vi "automatic_feeder.vi"() -> ()   [LabVIEW 2017]
panel:
  out "Boolean":bool
  out "Low  2":bool
  out "Ok  2":bool
  out "Full  2":bool
  out "Cup 2":dbl(slide) scale=0.0..3.0
  out "Tank 2":dbl(slide)=6.0 scale=0.0..3.0
  out "Lamp":bool
  in  "Thermometer":i32(slide) scale=0.0..100.0
  in  "Reset":bool
  in  "Lamp":bool
  in  "Stop":bool
  in  "?":bool
  out "Low":bool
  out "Ok":bool
  out "Full":bool
  out "Tank":dbl(slide)=6.0 scale=0.0..5.0
  out "Cup":dbl(slide) scale=0.0..5.0
  out "OK Button":bool
  in  "Clock":i32(knob)=1 min=1 max=12 scale=1.0..12.0
  # "EMPTY/FILL"
  # "FOOD"
  # "WATER"
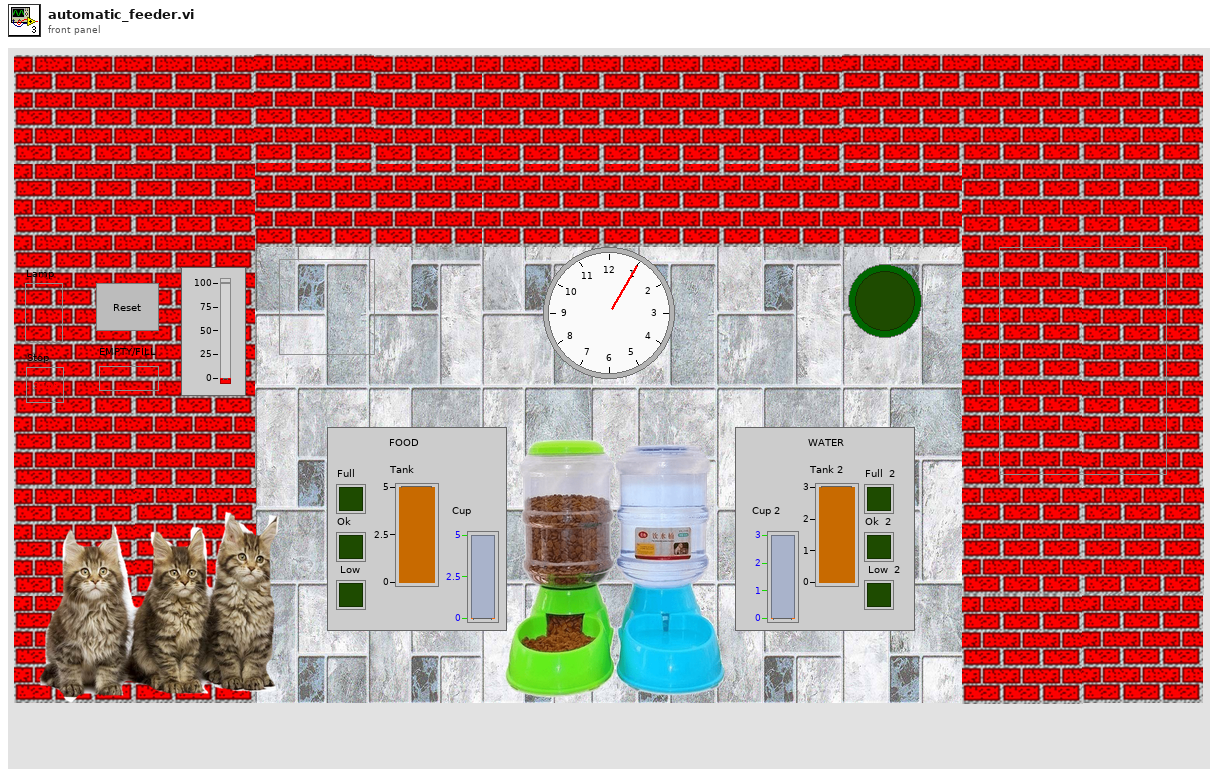
[diagram p1: front panel]
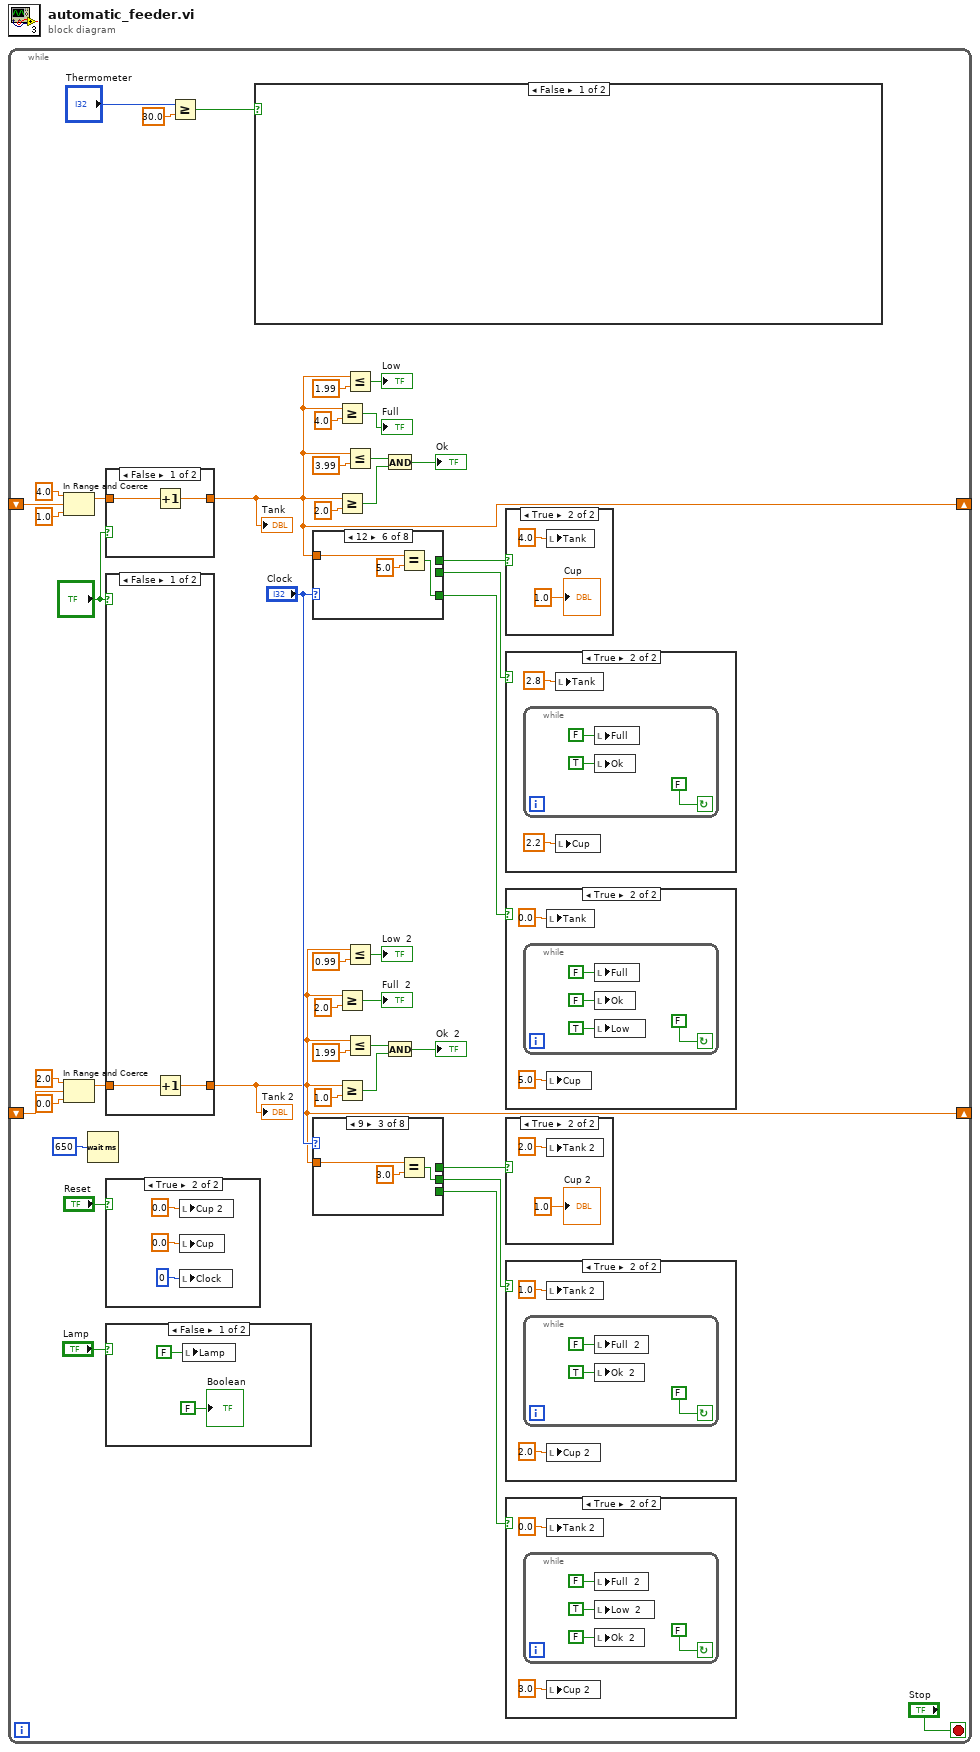
[diagram p0: block diagram]
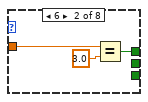
[diagram p6: hidden frame]
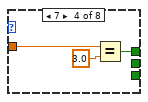
[diagram p7: hidden frame]
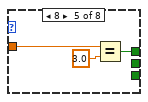
[diagram p8: hidden frame]
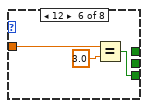
[diagram p9: hidden frame]
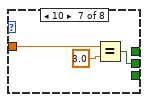
[diagram p10: hidden frame]
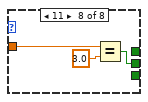
[diagram p11: hidden frame]
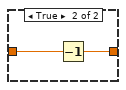
[diagram p12: hidden frame]
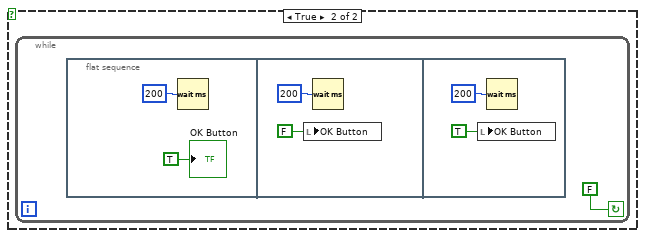
[diagram p13: hidden frame]
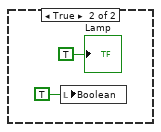
[diagram p14: hidden frame]
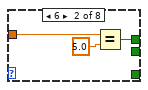
[diagram p19: hidden frame]
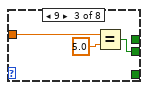
[diagram p20: hidden frame]
diagram:
  n1 = while {
    shift-right: [w27] -> _
    shift-left: _ -> [w30]
    shift-right: [w8] -> _
    shift-left: _ -> [w19]
    stop <- "Stop" stop-if-true
    n2 = In Range and Coerce(upper limit=4.0, x=w30, lower limit=1.0) -> (coerced(x)=w40:dbl)  [unwired: 1 out]
    n3 = In Range and Coerce(upper limit=2.0, x=w19, lower limit=0.0) -> (coerced(x)=w16:dbl)  [unwired: 1 out]
    n4 = Wait (ms)(milliseconds to wait=u32 650) -> ()  [unwired: 1 out]
    n5 = case shown="False" "?" {
      tunnel: w40 -> [w131 w133]
      tunnel: [w130 w132] -> w27
      frame False {
        n6 = Increment(x=w131) -> (x+1=w130:dbl)
      }
      frame True {
        n7 = Decrement(x=w133) -> (x-1=w132:dbl)
      }
    }
    "Tank" <- w27
    n8 = case shown="False" "?" {
      tunnel: w16 -> [w79 w81]
      tunnel: [w78 w80] -> w8
      frame False {
        n9 = Increment(x=w79) -> (x+1=w78:dbl)
      }
      frame True {
        n10 = Decrement(x=w81) -> (x-1=w80:dbl)
      }
    }
    "Tank 2" <- w8
    n11 = case shown="True" "Reset" {
      frame False {
      }
      frame True {
        n12 = local write "Cup 2"(0.0 ("Cup 2")) -> ()
        n13 = local write "Cup"(0.0 ("Tank")) -> ()
        n14 = local write "Clock"(0 ("Gauge")) -> ()
      }
    }
    n15 = case shown="False" "Lamp" {
      frame False {
        n16 = local write "Lamp"(FALSE ("Lamp")) -> ()
        "Boolean" <- FALSE ("Boolean")
      }
      frame True {
        n17 = local write "Boolean"(TRUE ("Boolean")) -> ()
        "Lamp" <- TRUE
      }
    }
    n18 = Greater Or Equal?(x="Thermometer", y=30.0) -> (x >= y?=w22:bool)
    n19 = case shown="False" w22 {
      frame False {
      }
      frame True {
        n20 = while {
          stop <- FALSE continue-if-true
          n21 = flat-sequence {
            frame #0 {
              n22 = Wait (ms)(milliseconds to wait=u32 200) -> ()  [unwired: 1 out]
              "OK Button" <- TRUE ("OK Button")
            }
            frame #1 {
              n23 = local write "OK Button"(FALSE ("OK Button")) -> ()
              n24 = Wait (ms)(milliseconds to wait=u32 200) -> ()  [unwired: 1 out]
            }
            frame #2 {
              n25 = local write "OK Button"(TRUE ("OK Button")) -> ()
              n26 = Wait (ms)(milliseconds to wait=u32 200) -> ()  [unwired: 1 out]
            }
          }
        }
      }
    }
    n27 = case shown="12" "Clock" {
      tunnel: [_ w108 _ w113 w117 _ _ _] -> w28
      tunnel: w27 -> [_ w107 w111 w114 w116 w120 w123 w126]
      tunnel: [_ _ w110 _ _ _ w122 w125] -> w25
      tunnel: [_ _ _ _ _ w119 _ _] -> w24
      frame 0, Default {
      }
      frame 6 {
        n28 = Equal?(x=w107, y=5.0) -> (x = y?=w108:bool)
      }
      frame 9 {
        n29 = Equal?(x=w111, y=5.0) -> (x = y?=w110:bool)
      }
      frame 7 {
        n30 = Equal?(x=w114, y=5.0) -> (x = y?=w113:bool)
      }
      frame 8 {
        n31 = Equal?(x=w116, y=5.0) -> (x = y?=w117:bool)
      }
      frame 12 {
        n32 = Equal?(x=w120, y=5.0) -> (x = y?=w119:bool)
      }
      frame 10 {
        n33 = Equal?(x=w123, y=5.0) -> (x = y?=w122:bool)
      }
      frame 11 {
        n34 = Equal?(x=w126, y=5.0) -> (x = y?=w125:bool)
      }
    }
    n35 = case shown="9" "Clock" {
      tunnel: [_ w58 _ w63 w67 _ _ _] -> w1
      tunnel: w8 -> [_ w57 w61 w64 w66 w70 w73 w76]
      tunnel: [_ _ w60 _ _ _ w72 w75] -> w7
      tunnel: [_ _ _ _ _ w69 _ _] -> w2
      frame 0, Default {
      }
      frame 6 {
        n36 = Equal?(x=w57, y=3.0) -> (x = y?=w58:bool)
      }
      frame 9 {
        n37 = Equal?(x=w61, y=3.0) -> (x = y?=w60:bool)
      }
      frame 7 {
        n38 = Equal?(x=w64, y=3.0) -> (x = y?=w63:bool)
      }
      frame 8 {
        n39 = Equal?(x=w66, y=3.0) -> (x = y?=w67:bool)
      }
      frame 12 {
        n40 = Equal?(x=w70, y=3.0) -> (x = y?=w69:bool)
      }
      frame 10 {
        n41 = Equal?(x=w73, y=3.0) -> (x = y?=w72:bool)
      }
      frame 11 {
        n42 = Equal?(x=w76, y=3.0) -> (x = y?=w75:bool)
      }
    }
    n43 = Greater Or Equal?(x=w27, y=4.0) -> (x >= y?=→"Full":bool)
    n44 = Greater Or Equal?(x=w27, y=2.0) -> (x >= y?=w37:bool)
    n45 = Greater Or Equal?(x=w8, y=2.0) -> (x >= y?=→"Full  2":bool)
    n46 = Greater Or Equal?(x=w8, y=1.0) -> (x >= y?=w13:bool)
    n47 = Less Or Equal?(x=w27, y=1.99) -> (x <= y?=→"Low":bool)
    n48 = Less Or Equal?(x=w27, y=3.99) -> (x <= y?=w35:bool)
    n49 = Less Or Equal?(x=w8, y=0.99) -> (x <= y?=→"Low  2":bool)
    n50 = Less Or Equal?(x=w8, y=1.99) -> (x <= y?=w14:bool)
    n51 = And(x=w35, y=w37) -> (x .and. y?=→"Ok":bool)
    n52 = And(x=w14, y=w13) -> (x .and. y?=→"Ok  2":bool)
    n53 = case shown="True" w28 {
      frame False {
      }
      frame True {
        n54 = local write "Tank"(4.0 ("x")) -> ()
        "Cup" <- 1.0 ("x")
      }
    }
    n55 = case shown="True" w25 {
      frame False {
      }
      frame True {
        n56 = while {
          stop <- FALSE continue-if-true
          n57 = local write "Full"(FALSE ("Full")) -> ()
          n58 = local write "Ok"(TRUE ("OK")) -> ()
        }
        n59 = local write "Tank"(2.8 ("x")) -> ()
        n60 = local write "Cup"(2.2 ("x")) -> ()
      }
    }
    n61 = case shown="True" w24 {
      frame False {
      }
      frame True {
        n62 = while {
          stop <- FALSE continue-if-true
          n63 = local write "Full"(FALSE ("Full")) -> ()
          n64 = local write "Ok"(FALSE ("OK")) -> ()
          n65 = local write "Low"(TRUE ("Low level")) -> ()
        }
        n66 = local write "Tank"(0.0 ("x")) -> ()
        n67 = local write "Cup"(5.0 ("x")) -> ()
      }
    }
    n68 = case shown="True" w1 {
      frame False {
      }
      frame True {
        n69 = local write "Tank 2"(2.0 ("Tank 2")) -> ()
        "Cup 2" <- 1.0 ("Cup 2")
      }
    }
    n70 = case shown="True" w7 {
      frame False {
      }
      frame True {
        n71 = while {
          stop <- FALSE continue-if-true
          n72 = local write "Full  2"(FALSE ("Full  2")) -> ()
          n73 = local write "Ok  2"(TRUE ("Ok  2")) -> ()
        }
        n74 = local write "Tank 2"(1.0 ("Tank 2")) -> ()
        n75 = local write "Cup 2"(2.0 ("Cup 2")) -> ()
      }
    }
    n76 = case shown="True" w2 {
      frame False {
      }
      frame True {
        n77 = while {
          stop <- FALSE continue-if-true
          n78 = local write "Full  2"(FALSE ("Full  2")) -> ()
          n79 = local write "Low  2"(TRUE ("Ok  2")) -> ()
          n80 = local write "Ok  2"(FALSE ("Ok  2")) -> ()
        }
        n81 = local write "Tank 2"(0.0 ("Tank 2")) -> ()
        n82 = local write "Cup 2"(3.0 ("Cup 2")) -> ()
      }
    }
  }
